vi "Get Used J1939 Addresses.vi"(8 "error in (no error)":errorcluster, 11 "Node Ptr":u64) -> (0 "error out":errorcluster, 2 "Nodes":T2[](array[typedef]) {"Name" format="%.0x"}, 3 "Item Ref out":T1 format="%.0x")   [LabVIEW 2019, in "J1939 Addon System Explorer.lvlib"]
uses:
  J1939 Addon System Explorer.lvlib
  Addon Shared/Types/Monitor Settings.ctl
  <vilib>/NI VeriStand/Custom Device API/Custom Device Item Ref.ctl
  <vilib>/NI VeriStand/Custom Device Tools/Custom Device Utility Library/Search Direction.ctl
  Addon Shared/SubVIs/Constants.vi
  <vilib>/NI VeriStand/Custom Device Tools/Custom Device Utility Library/NI VeriStand - Search for Item by GUID.vi
  <vilib>/NI VeriStand/Custom Device Tools/Custom Device Utility Library/NI VeriStand - Search for All Items by GUID.vi
  Addon Shared/J1939 Addon Shared.lvlib
  <vilib>/NI VeriStand/Custom Device Tools/Custom Device Utility Library/Custom Device Utility Library.lvlib
  <vilib>/NI VeriStand/Custom Device API/Custom Device API.lvlib
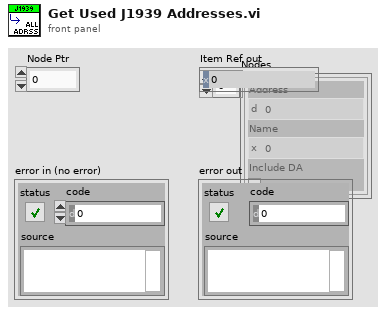
[diagram p1: front panel]
types:
  T1 = typedef "Custom Device API.lvlib/Custom Device Item Ref.ctl" = u64
  T2 = typedef "J1939 Addon Shared.lvlib/Monitor Settings.ctl" = cluster{"Address":u8, "Name":u64, "Include DA":bool}
  T3 = typedef "Custom Device Utility Library.lvlib/Search Direction.ctl" = enum16{"Down", "Up"}
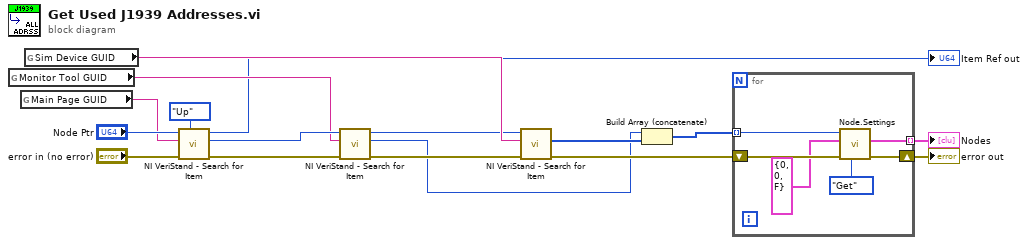
[diagram p0: block diagram]
diagram:
  n1 = global read "Constants.vi" "Monitor Tool GUID"() -> (w7:string)
  n2 = global read "Constants.vi" "Main Page GUID"() -> (w11:string)
  n3 = global read "Constants.vi" "Sim Device GUID"() -> (w15:string)
  n4 = call-poly <vilib>:"NI VeriStand - Search for Item.vi"("Direction (Down)"=Search_Direction."Up", "error in"="error in (no error)", "Item GUID"=w11, "Section Ref in"="Node Ptr") -> ("error out"=w9:errorcluster, "Item Ref"=w10:T1, "Section Ref out"=→"Item Ref out":T1)  [unwired: 4 in, 1 out]
  n5 = call-poly <vilib>:"NI VeriStand - Search for Item.vi"("error in"=w9, "Item GUID"=w7, "Section Ref in"=w10) -> ("error out"=w8:errorcluster, "Item Ref"=w5:T1, "Section Ref out"=w3:T1)  [unwired: 5 in, 1 out]
  n6 = call-poly <vilib>:"NI VeriStand - Search for Item.vi"("error in"=w8, "Item GUID"=w15, "Section Ref in"=w3) -> ("error out"=w16:errorcluster, "Item Refs"=w6:T1[])  [unwired: 5 in, 2 out]
  n7 = Build Array (concatenate)(w5, w6) -> (w4:T1[])
  n8 = for {
    shift-right: [w22] -> w17
    shift-left: w16 -> [w23]
    tunnel: w4 -> [w21] mode=indexing
    tunnel: [w19] -> w1 mode=indexing
    n9 = call "Node.Settings.vi"("Action"=enum8{"Get", "Set"}."Get", "error in (no error)"=w23, "Node.Settings"=T2 {"Address"=0, "Name"=0, "Include DA"=FALSE} ("J1939 XNET Settings"), "Item Ref in"=w21) -> ("error out"=w22:errorcluster, "Node.Settings"=w19:T2)  [unwired: 5 in, 1 out]
  }
  "Nodes" <- w1
  "error out" <- w17
